vi "Unrock_Data_To_Unrock_Cluster.vi"(1 "Cluster67":T4) -> (0 "Cluster8":T1)   [LabVIEW 2019]
uses:
  Unrock_Data.ctl
  Unrock_Cluster.ctl
  Test_load.ctl
  Hardness_test.ctl
  TEST.lvclass
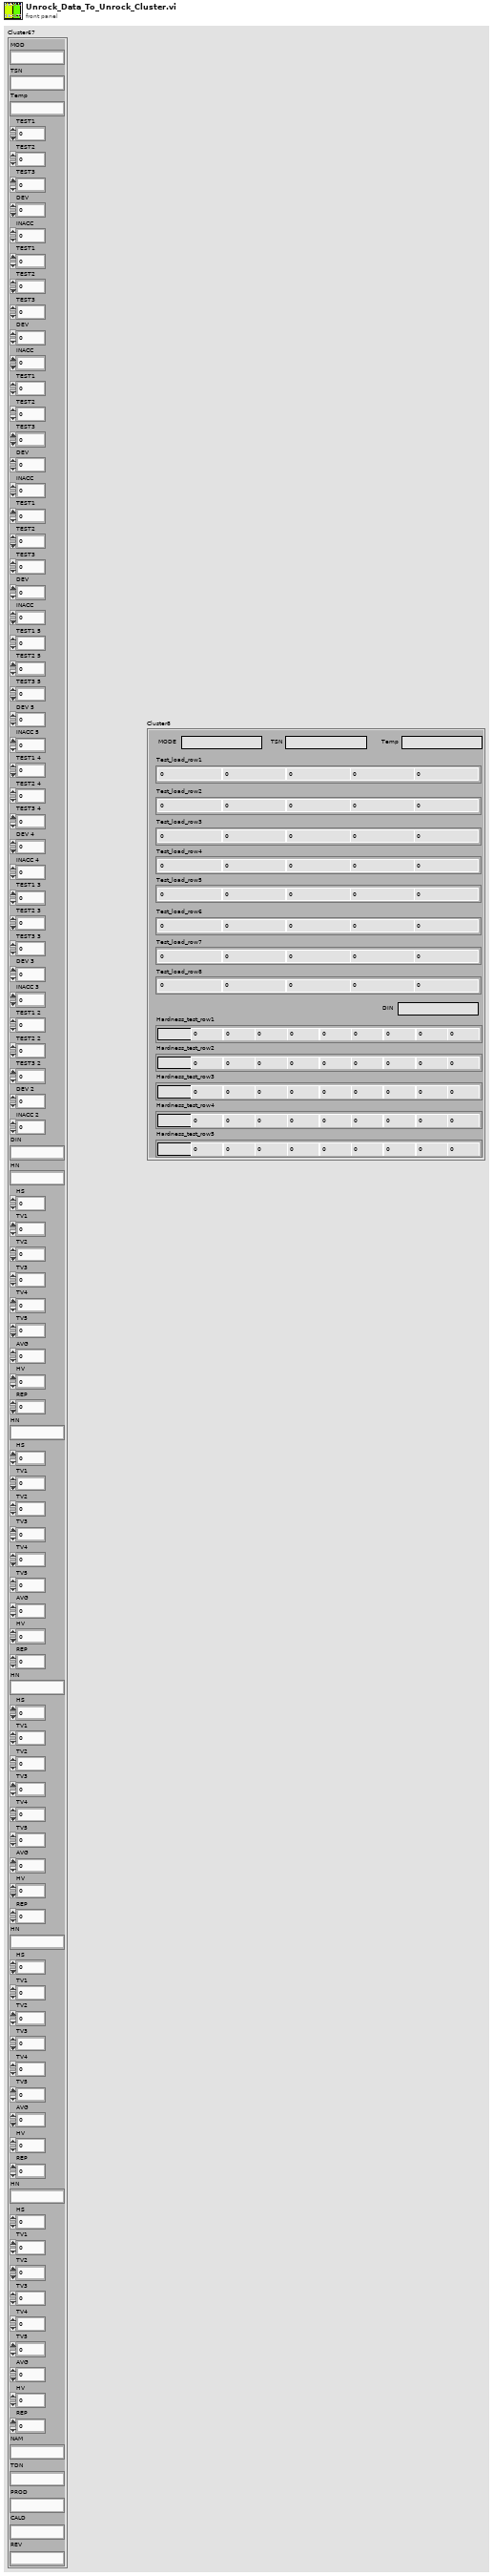
[diagram p1: front panel]
types:
  T1 = typedef "TEST.lvclass/Unrock_Cluster.ctl" = cluster{"MODE":string, "TSN":string, "Temp":string, "Test_load_row1":T2, "Test_load_row2":T2, "Test_load_row3":T2, "Test_load_row4":T2, "Test_load_row5":T2, "Test_load_row6":T2, "Test_load_row7":T2, "Test_load_row8":T2, "DIN":string, "Hardness_test_row1":T3, "Hardness_test_row2":T3, "Hardness_test_row3":T3, "Hardness_test_row4":T3, "Hardness_test_row5":T3}
  T2 = typedef "TEST.lvclass/Test_load.ctl" = cluster{"TEST1":sgl, "TEST2":sgl, "TEST3":sgl, "DEV":sgl, "INACC":sgl}
  T3 = typedef "TEST.lvclass/Hardness_test.ctl" = cluster{"HN":string, "HS":sgl, "TV1":sgl, "TV2":sgl, "TV3":sgl, "TV4":sgl, "TV5":sgl, "AVG":sgl, "HV":sgl, "REP":sgl}
  T4 = typedef "TEST.lvclass/Unrock_Data.ctl" = cluster{"MOD":string, "TSN":string, "Temp":string, "TEST1":sgl, "TEST2":sgl, "TEST3":sgl, "DEV":sgl, "INACC":sgl, "TEST1":sgl, "TEST2":sgl, "TEST3":sgl, "DEV":sgl, "INACC":sgl, "TEST1":sgl, "TEST2":sgl, "TEST3":sgl, "DEV":sgl, "INACC":sgl, "TEST1":sgl, "TEST2":sgl, "TEST3":sgl, "DEV":sgl, "INACC":sgl, "TEST1 5":sgl, "TEST2 5":sgl, "TEST3 5":sgl, "DEV 5":sgl, "INACC 5":sgl, "TEST1 4":sgl, "TEST2 4":sgl, "TEST3 4":sgl, "DEV 4":sgl, "INACC 4":sgl, "TEST1 3":sgl, "TEST2 3":sgl, "TEST3 3":sgl, "DEV 3":sgl, "INACC 3":sgl, "TEST1 2":sgl, "TEST2 2":sgl, "TEST3 2":sgl, "DEV 2":sgl, "INACC 2":sgl, "DIN":string, "HN":string, "HS":sgl, "TV1":sgl, "TV2":sgl, "TV3":sgl, "TV4":sgl, "TV5":sgl, "AVG":sgl, "HV":sgl, "REP":sgl, "HN":string, "HS":sgl, "TV1":sgl, "TV2":sgl, "TV3":sgl, "TV4":sgl, "TV5":sgl, "AVG":sgl, "HV":sgl, "REP":sgl, "HN":string, "HS":sgl, "TV1":sgl, "TV2":sgl, "TV3":sgl, "TV4":sgl, "TV5":sgl, "AVG":sgl, "HV":sgl, "REP":sgl, "HN":string, "HS":sgl, "TV1":sgl, "TV2":sgl, "TV3":sgl, "TV4":sgl, "TV5":sgl, "AVG":sgl, "HV":sgl, "REP":sgl, "HN":string, "HS":sgl, "TV1":sgl, "TV2":sgl, "TV3":sgl, "TV4":sgl, "TV5":sgl, "AVG":sgl, "HV":sgl, "REP":sgl, "NAM":string, "TDN":string, "PROD":string, "CALD":string, "REV":string}
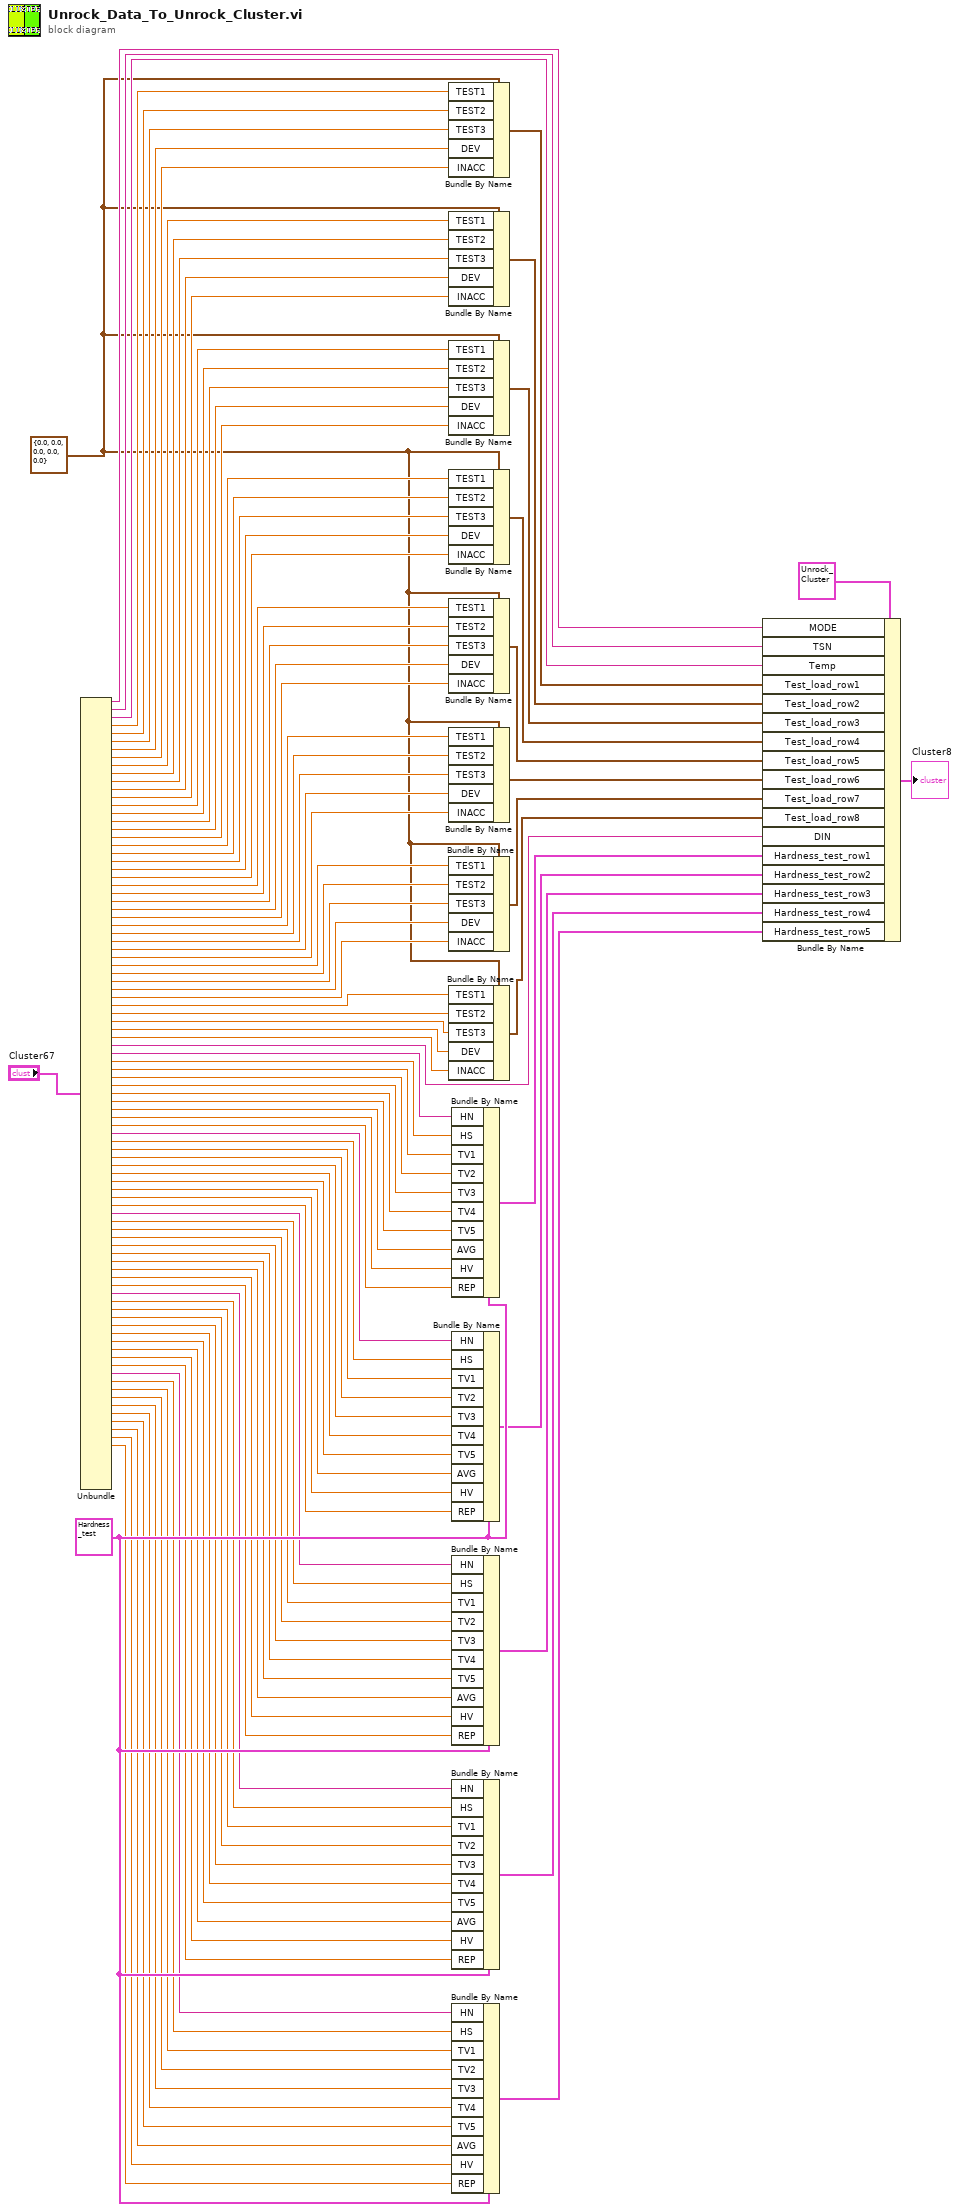
[diagram p0: block diagram]
diagram:
  w111 = T3 {"HN"="", "HS"=0.0, "TV1"=0.0, "TV2"=0.0, "TV3"=0.0, "TV4"=0.0, "TV5"=0.0, "AVG"=0.0, "HV"=0.0, "REP"=0.0} ("Hardness_test")
  w1 = T2 {"TEST1"=0.0, "TEST2"=0.0, "TEST3"=0.0, "DEV"=0.0, "INACC"=0.0} ("Test_load")
  n1 = Unbundle("Cluster67") -> ("MOD"=w97:string, "TSN"=w99:string, "Temp"=w98:string, "TEST1"=w96:sgl, "TEST2"=w95:sgl, "TEST3"=w94:sgl, "DEV"=w93:sgl, "INACC"=w92:sgl, "TEST1"=w91:sgl, "TEST2"=w90:sgl, "TEST3"=w89:sgl, "DEV"=w88:sgl, "INACC"=w87:sgl, "TEST1"=w86:sgl, "TEST2"=w85:sgl, "TEST3"=w84:sgl, "DEV"=w83:sgl, "INACC"=w82:sgl, "TEST1"=w81:sgl, "TEST2"=w80:sgl, "TEST3"=w79:sgl, "DEV"=w78:sgl, "INACC"=w77:sgl, "TEST1 5"=w25:sgl, "TEST2 5"=w24:sgl, "TEST3 5"=w23:sgl, "DEV 5"=w22:sgl, "INACC 5"=w21:sgl, "TEST1 4"=w20:sgl, "TEST2 4"=w19:sgl, "TEST3 4"=w18:sgl, "DEV 4"=w17:sgl, "INACC 4"=w16:sgl, "TEST1 3"=w15:sgl, "TEST2 3"=w14:sgl, "TEST3 3"=w13:sgl, "DEV 3"=w12:sgl, "INACC 3"=w11:sgl, "TEST1 2"=w10:sgl, "TEST2 2"=w9:sgl, "TEST3 2"=w8:sgl, "DEV 2"=w7:sgl, "INACC 2"=w6:sgl, "DIN"=w66:string, "HN"=w76:string, "HS"=w75:sgl, "TV1"=w74:sgl, "TV2"=w73:sgl, "TV3"=w72:sgl, "TV4"=w71:sgl, "TV5"=w70:sgl, "AVG"=w69:sgl, "HV"=w68:sgl, "REP"=w67:sgl, "HN"=w65:string, "HS"=w64:sgl, "TV1"=w63:sgl, "TV2"=w62:sgl, "TV3"=w61:sgl, "TV4"=w60:sgl, "TV5"=w59:sgl, "AVG"=w58:sgl, "HV"=w57:sgl, "REP"=w56:sgl, "HN"=w55:string, "HS"=w54:sgl, "TV1"=w53:sgl, "TV2"=w52:sgl, "TV3"=w51:sgl, "TV4"=w50:sgl, "TV5"=w49:sgl, "AVG"=w48:sgl, "HV"=w47:sgl, "REP"=w46:sgl, "HN"=w45:string, "HS"=w44:sgl, "TV1"=w43:sgl, "TV2"=w42:sgl, "TV3"=w41:sgl, "TV4"=w40:sgl, "TV5"=w39:sgl, "AVG"=w38:sgl, "HV"=w37:sgl, "REP"=w36:sgl, "HN"=w35:string, "HS"=w34:sgl, "TV1"=w33:sgl, "TV2"=w32:sgl, "TV3"=w31:sgl, "TV4"=w30:sgl, "TV5"=w29:sgl, "AVG"=w28:sgl, "HV"=w27:sgl, "REP"=w26:sgl)  [unwired: 5 out]
  n2 = Bundle By Name(cluster=w1, "TEST1"=w96, "TEST2"=w95, "TEST3"=w94, "DEV"=w93, "INACC"=w92) -> (w109:T2)
  n3 = Bundle By Name(cluster=w1, "TEST1"=w91, "TEST2"=w90, "TEST3"=w89, "DEV"=w88, "INACC"=w87) -> (w108:T2)
  n4 = Bundle By Name(cluster=w1, "TEST1"=w86, "TEST2"=w85, "TEST3"=w84, "DEV"=w83, "INACC"=w82) -> (w107:T2)
  n5 = Bundle By Name(cluster=w1, "TEST1"=w81, "TEST2"=w80, "TEST3"=w79, "DEV"=w78, "INACC"=w77) -> (w105:T2)
  n6 = Bundle By Name(cluster=w1, "TEST1"=w25, "TEST2"=w24, "TEST3"=w23, "DEV"=w22, "INACC"=w21) -> (w5:T2)
  n7 = Bundle By Name(cluster=w1, "TEST1"=w20, "TEST2"=w19, "TEST3"=w18, "DEV"=w17, "INACC"=w16) -> (w4:T2)
  n8 = Bundle By Name(cluster=w1, "TEST1"=w15, "TEST2"=w14, "TEST3"=w13, "DEV"=w12, "INACC"=w11) -> (w3:T2)
  n9 = Bundle By Name(cluster=w1, "TEST1"=w10, "TEST2"=w9, "TEST3"=w8, "DEV"=w7, "INACC"=w6) -> (w2:T2)
  n10 = Bundle By Name(cluster=w111, "HN"=w76, "HS"=w75, "TV1"=w74, "TV2"=w73, "TV3"=w72, "TV4"=w71, "TV5"=w70, "AVG"=w69, "HV"=w68, "REP"=w67) -> (w104:T3)
  n11 = Bundle By Name(cluster=w111, "HN"=w65, "HS"=w64, "TV1"=w63, "TV2"=w62, "TV3"=w61, "TV4"=w60, "TV5"=w59, "AVG"=w58, "HV"=w57, "REP"=w56) -> (w103:T3)
  n12 = Bundle By Name(cluster=w111, "HN"=w55, "HS"=w54, "TV1"=w53, "TV2"=w52, "TV3"=w51, "TV4"=w50, "TV5"=w49, "AVG"=w48, "HV"=w47, "REP"=w46) -> (w102:T3)
  n13 = Bundle By Name(cluster=w111, "HN"=w45, "HS"=w44, "TV1"=w43, "TV2"=w42, "TV3"=w41, "TV4"=w40, "TV5"=w39, "AVG"=w38, "HV"=w37, "REP"=w36) -> (w101:T3)
  n14 = Bundle By Name(cluster=w111, "HN"=w35, "HS"=w34, "TV1"=w33, "TV2"=w32, "TV3"=w31, "TV4"=w30, "TV5"=w29, "AVG"=w28, "HV"=w27, "REP"=w26) -> (w100:T3)
  n15 = Bundle By Name(cluster=T1 {"MODE"="", "TSN"="", "Temp"="", "Test_load_row1"={"TEST1"=0.0, "TEST2"=0.0, "TEST3"=0.0, "DEV"=0.0, "INACC"=0.0}, "Test_load_row2"={"TEST1"=0.0, "TEST2"=0.0, "TEST3"=0.0, "DEV"=0.0, "INACC"=0.0}, "Test_load_row3"={"TEST1"=0.0, "TEST2"=0.0, "TEST3"=0.0, "DEV"=0.0, "INACC"=0.0}, "Test_load_row4"={"TEST1"=0.0, "TEST2"=0.0, "TEST3"=0.0, "DEV"=0.0, "INACC"=0.0}, "Test_load_row5"={"TEST1"=0.0, "TEST2"=0.0, "TEST3"=0.0, "DEV"=0.0, "INACC"=0.0}, "Test_load_row6"={"TEST1"=0.0, "TEST2"=0.0, "TEST3"=0.0, "DEV"=0.0, "INACC"=0.0}, "Test_load_row7"={"TEST1"=0.0, "TEST2"=0.0, "TEST3"=0.0, "DEV"=0.0, "INACC"=0.0}, "Test_load_row8"={"TEST1"=0.0, "TEST2"=0.0, "TEST3"=0.0, "DEV"=0.0, "INACC"=0.0}, "DIN"="", "Hardness_test_row1"={"HN"="", "HS"=0.0, "TV1"=0.0, "TV2"=0.0, "TV3"=0.0, "TV4"=0.0, "TV5"=0.0, "AVG"=0.0, "HV"=0.0, "REP"=0.0}, "Hardness_test_row2"={"HN"="", "HS"=0.0, "TV1"=0.0, "TV2"=0.0, "TV3"=0.0, "TV4"=0.0, "TV5"=0.0, "AVG"=0.0, "HV"=0.0, "REP"=0.0}, "Hardness_test_row3"={"HN"="", "HS"=0.0, "TV1"=0.0, "TV2"=0.0, "TV3"=0.0, "TV4"=0.0, "TV5"=0.0, "AVG"=0.0, "HV"=0.0, "REP"=0.0}, "Hardness_test_row4"={"HN"="", "HS"=0.0, "TV1"=0.0, "TV2"=0.0, "TV3"=0.0, "TV4"=0.0, "TV5"=0.0, "AVG"=0.0, "HV"=0.0, "REP"=0.0}, "Hardness_test_row5"={"HN"="", "HS"=0.0, "TV1"=0.0, "TV2"=0.0, "TV3"=0.0, "TV4"=0.0, "TV5"=0.0, "AVG"=0.0, "HV"=0.0, "REP"=0.0}} ("簇"), "MODE"=w97, "TSN"=w99, "Temp"=w98, "Test_load_row1"=w109, "Test_load_row2"=w108, "Test_load_row3"=w107, "Test_load_row4"=w105, "Test_load_row5"=w5, "Test_load_row6"=w4, "Test_load_row7"=w3, "Test_load_row8"=w2, "DIN"=w66, "Hardness_test_row1"=w104, "Hardness_test_row2"=w103, "Hardness_test_row3"=w102, "Hardness_test_row4"=w101, "Hardness_test_row5"=w100) -> (→"Cluster8":T1)
